vi "Logic_gates.vi"() -> ()   [LabVIEW 2026]
panel:
  in  "Boolean 4":bool
  in  "Boolean 3":bool
  in  "Boolean 2":bool
  in  "Boolean":bool
  out "XOR_M":bool
  in  "B":bool
  in  "A":bool
  out "XNOR":bool
  out "XOR":bool
  out "NOR":bool
  out "NAND":bool
  out "OR":bool
  out "AND":bool
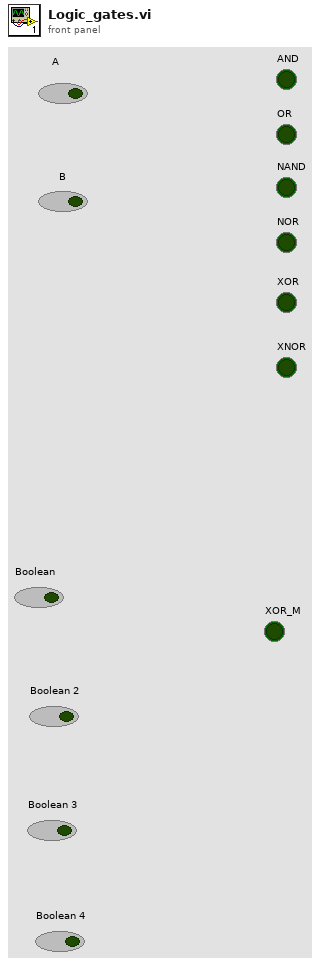
[diagram p1: front panel]
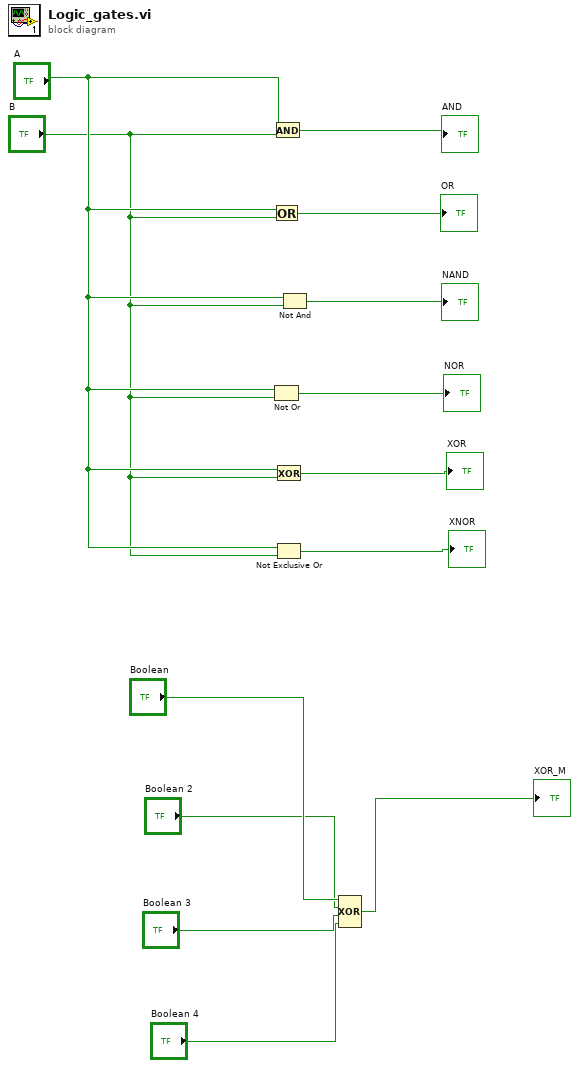
[diagram p0: block diagram]
diagram:
  n1 = Not Or(1:"B", 2:"A") -> (0:→"NOR":bool)
  n2 = Or(x="A", y="B") -> (x .or. y?=→"OR":bool)
  n3 = And(x="A", y="B") -> (x .and. y?=→"AND":bool)
  n4 = Exclusive Or(1:"B", 2:"A") -> (0:→"XOR":bool)
  n5 = Not Exclusive Or(1:"B", 2:"A") -> (0:→"XNOR":bool)
  n6 = Not And(1:"B", 2:"A") -> (0:→"NAND":bool)
  n7 = Compound Arithmetic op=XOR("Boolean", "Boolean 2", "Boolean 3", "Boolean 4") -> (→"XOR_M":bool)
